vi "Get Plugin Paths.vi"(8 "error in":errorcluster, 11 "measurement in":refnum<class "Continuous Counting Measurement.lvclass">) -> (0 "error out":errorcluster, 2 "plugin paths":T1, 3 "measurement out":refnum<class "Continuous Counting Measurement.lvclass">)   [LabVIEW 2021, in "MeasurementServerTests.lvlib" / "Measurement Service Tests.lvlib" / "Continuous Counting Measurement.lvclass"]
uses:
  Continuous Counting Measurement.lvclass
  Runtime/Measurements/Measurement Plugin Service/Plugin Paths.ctl
  _Get Type Specializations.vi
  _Get Measurement Details.vi
  _Reentrant Measurement.vi
  _Get UI Details.vi
  Measurement Configuration.ctl
  Measurement Results.ctl
  _Non-Reentrant Measurement.vi
  Runtime/Measurements/Measurement Plugin Service/Measurement Plugin Service.lvclass
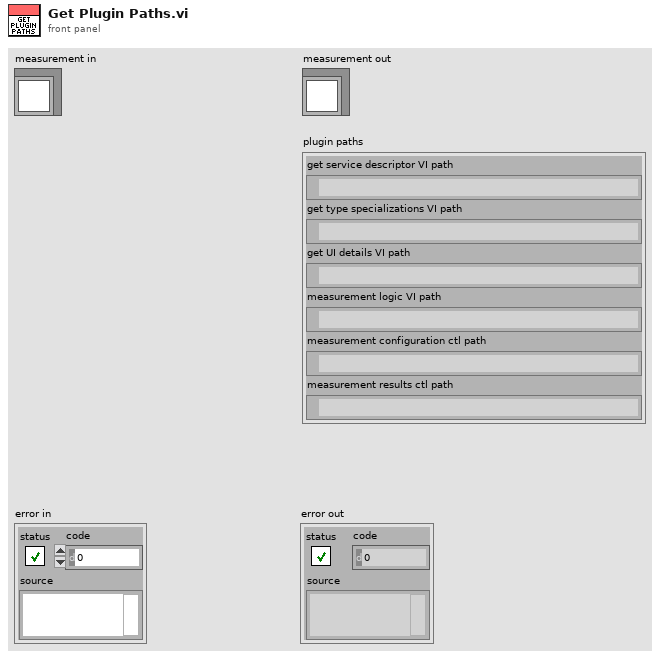
[diagram p1: front panel]
types:
  T1 = typedef "NI Measurement Plug-In SDK.lvlib/Measurement Plugin Service.lvclass/Plugin Paths.ctl" = cluster{"get service descriptor VI path":path, "get type specializations VI path":path, "get UI details VI path":path, "measurement logic VI path":path, "measurement configuration ctl path":path, "measurement results ctl path":path}
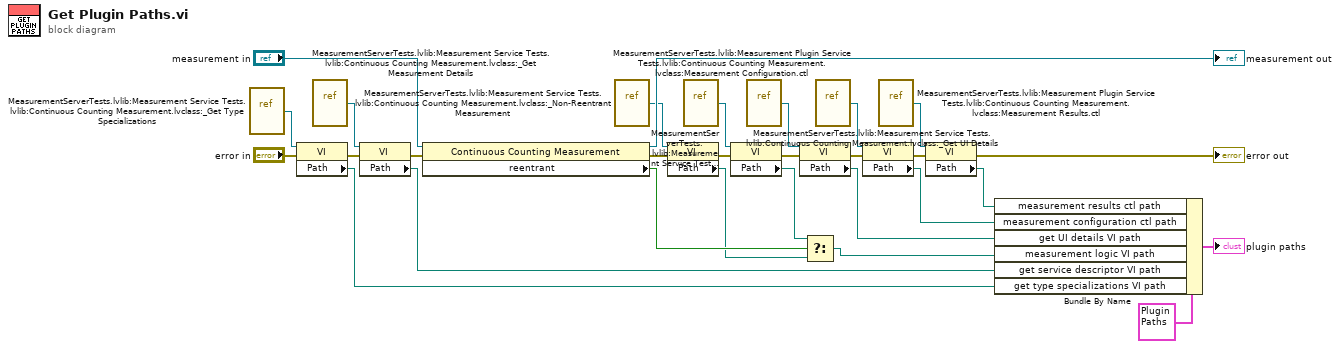
[diagram p0: block diagram]
diagram:
  n1 = vi-ref "MeasurementServerTests.lvlib:Measurement Service Tests.lvlib:Continuous Counting Measurement.lvclass:_Get Type Specializations.vi"() -> (w17:refnum<vi>)
  n2 = property class="VI"(reference=w17, error in="error in") -> (error out=w27:errorcluster, "Path"=w26:path)  [unwired: 1 out]
  n3 = vi-ref "MeasurementServerTests.lvlib:Measurement Service Tests.lvlib:Continuous Counting Measurement.lvclass:_Get Measurement Details.vi"() -> (w16:refnum<vi>)
  n4 = property class="VI"(reference=w16, error in=w27) -> (error out=w2:errorcluster, "Path"=w25:path)  [unwired: 1 out]
  n5 = property class="Continuous Counting Measurement"(reference="measurement in", error in=w2) -> (reference out=→"measurement out":refnum<class "Continuous Counting Measurement.lvclass">, error out=w1:errorcluster, "reentrant"=w8:bool)
  n6 = vi-ref "MeasurementServerTests.lvlib:Measurement Service Tests.lvlib:Continuous Counting Measurement.lvclass:_Non-Reentrant Measurement.vi"() -> (w9:refnum<vi>)
  n7 = property class="VI"(reference=w9, error in=w1) -> (error out=w6:errorcluster, "Path"=w5:path)  [unwired: 1 out]
  n8 = vi-ref "MeasurementServerTests.lvlib:Measurement Service Tests.lvlib:Continuous Counting Measurement.lvclass:_Reentrant Measurement.vi"() -> (w15:refnum<vi>)
  n9 = property class="VI"(reference=w15, error in=w6) -> (error out=w3:errorcluster, "Path"=w7:path)  [unwired: 1 out]
  n10 = vi-ref "MeasurementServerTests.lvlib:Measurement Service Tests.lvlib:Continuous Counting Measurement.lvclass:_Get UI Details.vi"() -> (w14:refnum<vi>)
  n11 = property class="VI"(reference=w14, error in=w3) -> (error out=w29:errorcluster, "Path"=w24:path)  [unwired: 1 out]
  n12 = Select(t=w7, s=w8, f=w5) -> (s? t:f=w4:path)
  n13 = vi-ref "MeasurementServerTests.lvlib:Measurement Plugin Service Tests.lvlib:Continuous Counting Measurement.lvclass:Measurement Configuration.ctl"() -> (w12:refnum<vi>)
  n14 = property class="VI"(reference=w12, error in=w29) -> (error out=w28:errorcluster, "Path"=w23:path)  [unwired: 1 out]
  n15 = vi-ref "MeasurementServerTests.lvlib:Measurement Plugin Service Tests.lvlib:Continuous Counting Measurement.lvclass:Measurement Results.ctl"() -> (w13:refnum<vi>)
  n16 = property class="VI"(reference=w13, error in=w28) -> (error out=→"error out":errorcluster, "Path"=w22:path)  [unwired: 1 out]
  n17 = Bundle By Name(cluster=T1 {"get service descriptor VI path"=path "", "get type specializations VI path"=path "", "get UI details VI path"=path "", "measurement logic VI path"=path "", "measurement configuration ctl path"=path "", "measurement results ctl path"=path ""} ("plugin paths"), "measurement results ctl path"=w22, "measurement configuration ctl path"=w23, "get UI details VI path"=w24, "measurement logic VI path"=w4, "get service descriptor VI path"=w25, "get type specializations VI path"=w26) -> (→"plugin paths":T1)
